vi "NI 9263_task.vi"(8 "error in":errorcluster, 11 "MODULE NAME":string="CDR_AO1") -> (0 "error out":errorcluster, 3 "task out":refnum<k21>)   [LabVIEW 2019]
uses:
  <vilib>/DAQmx/create/channels.llb/DAQmx Create Channel (AO-Voltage-Basic).vi
  <resource>/objmgr/daqmx.rc
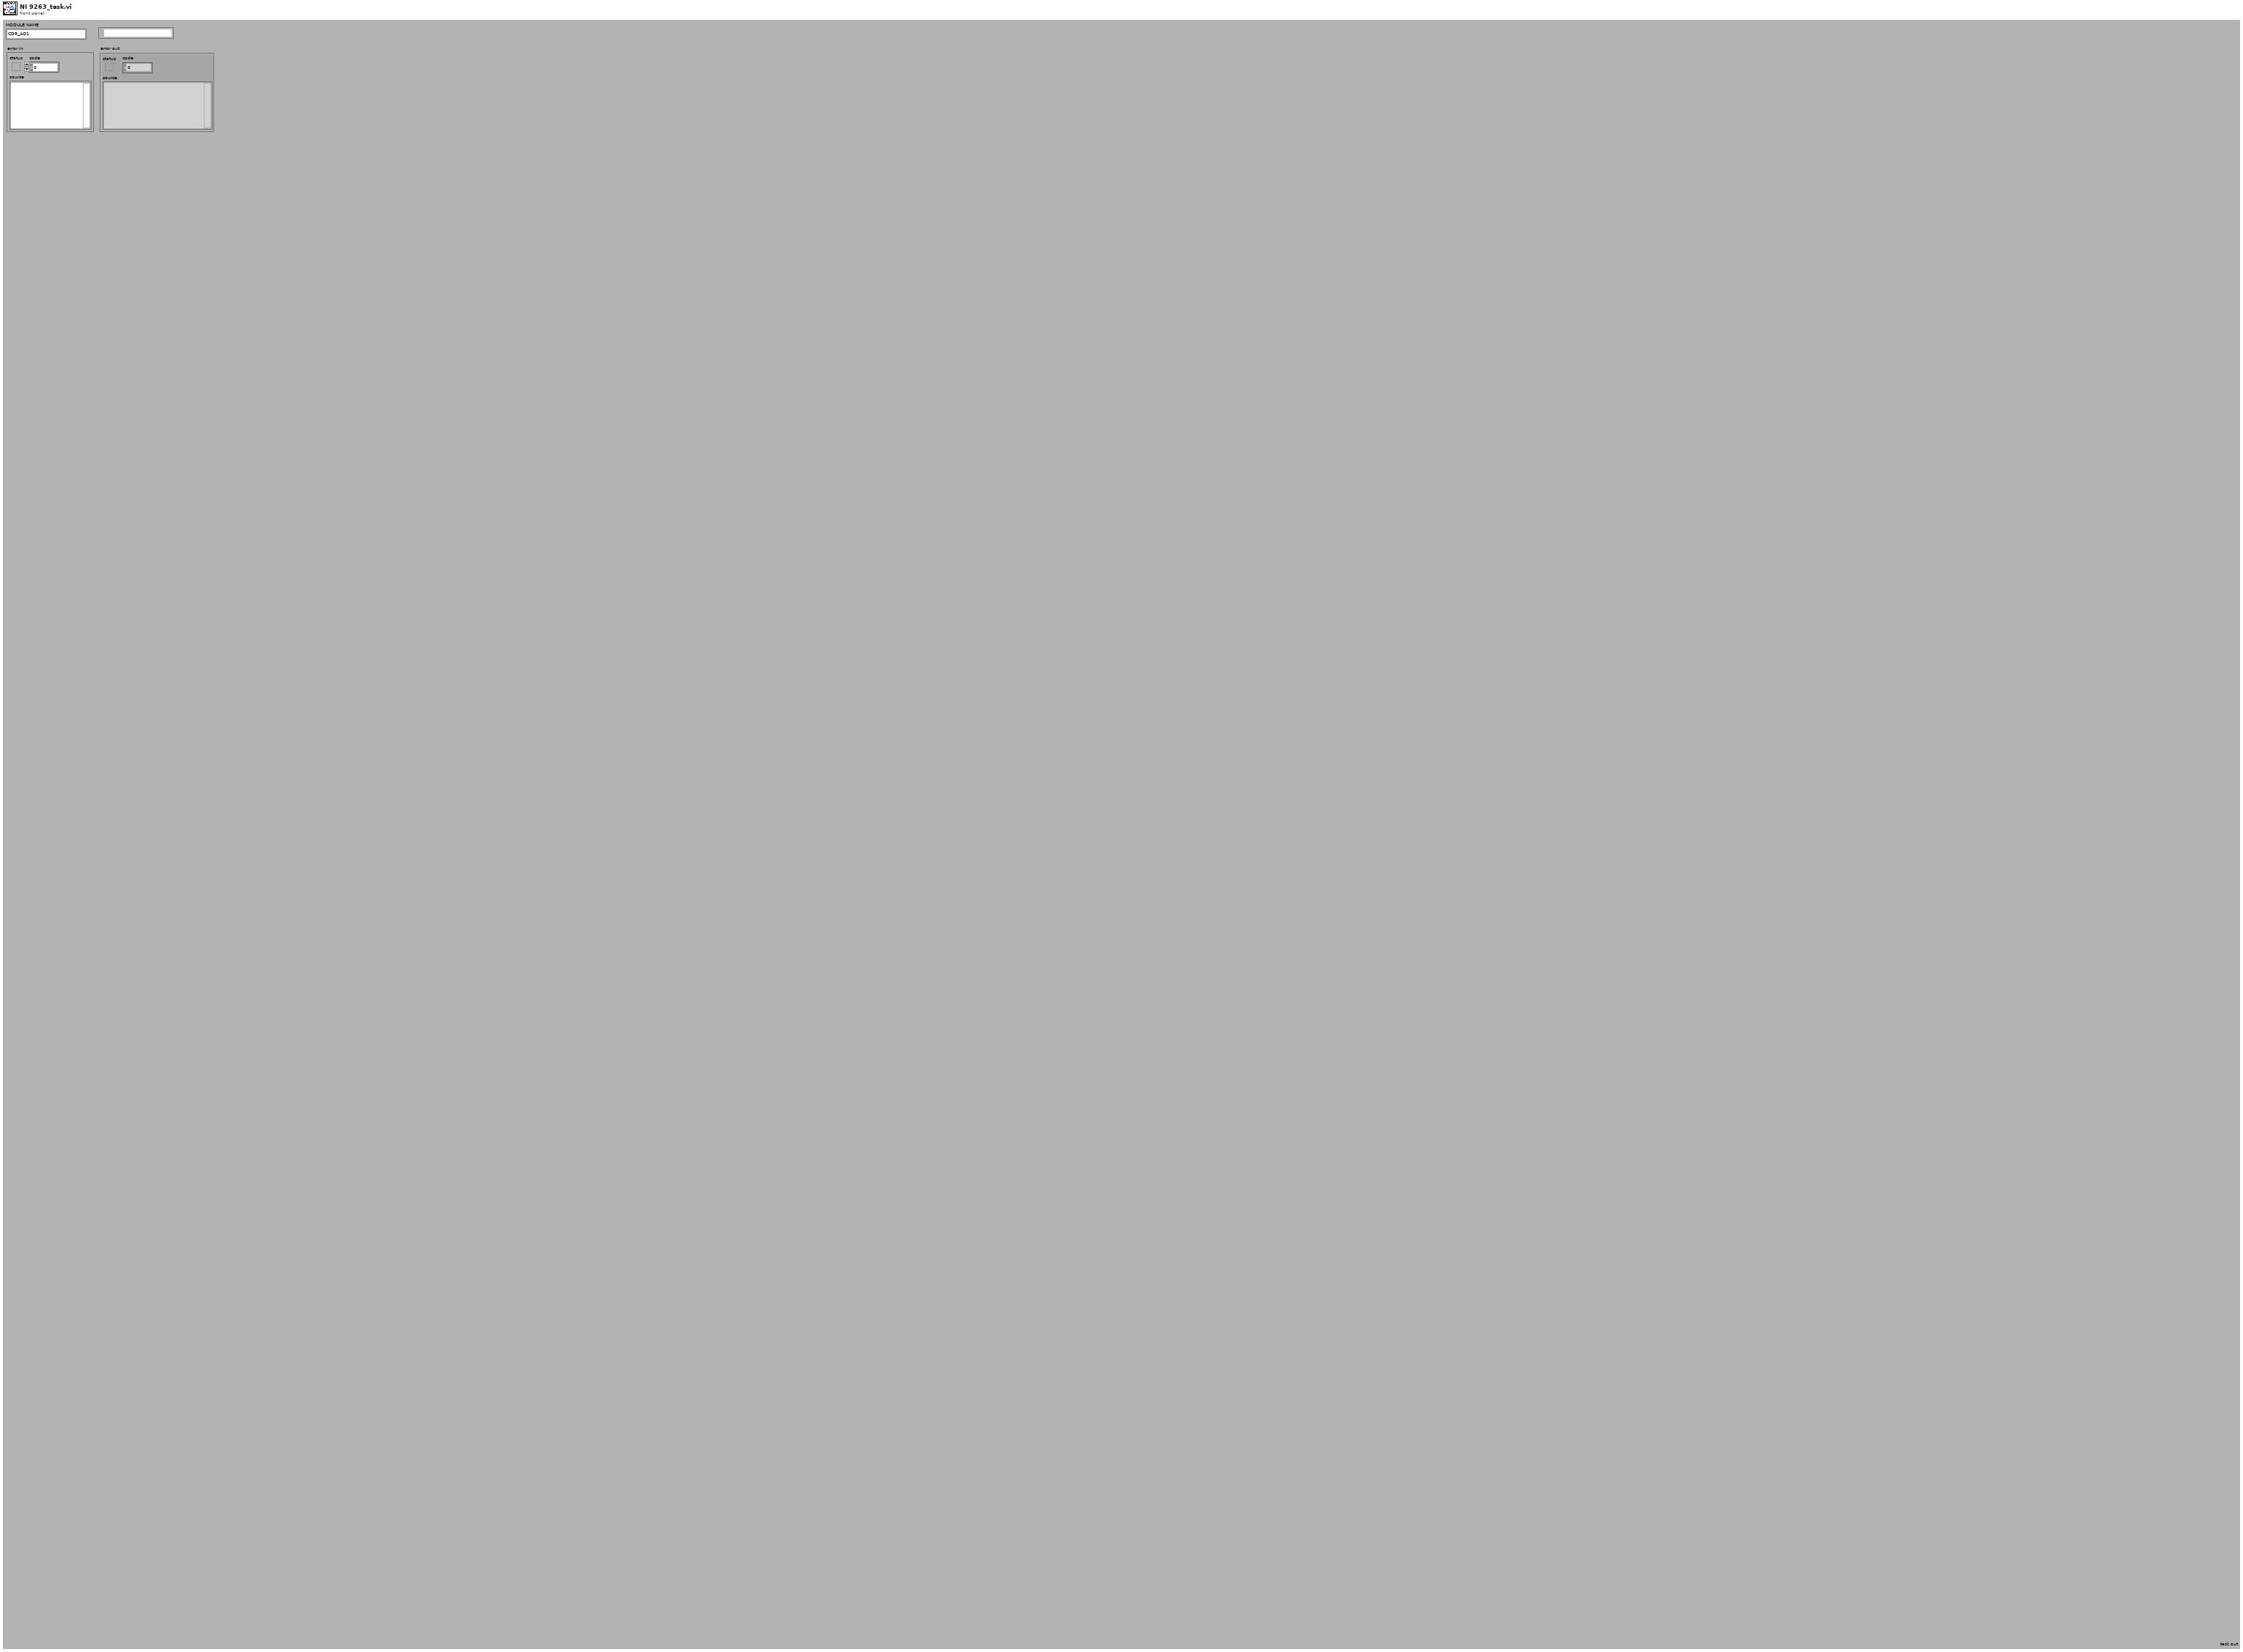
[diagram p1: front panel]
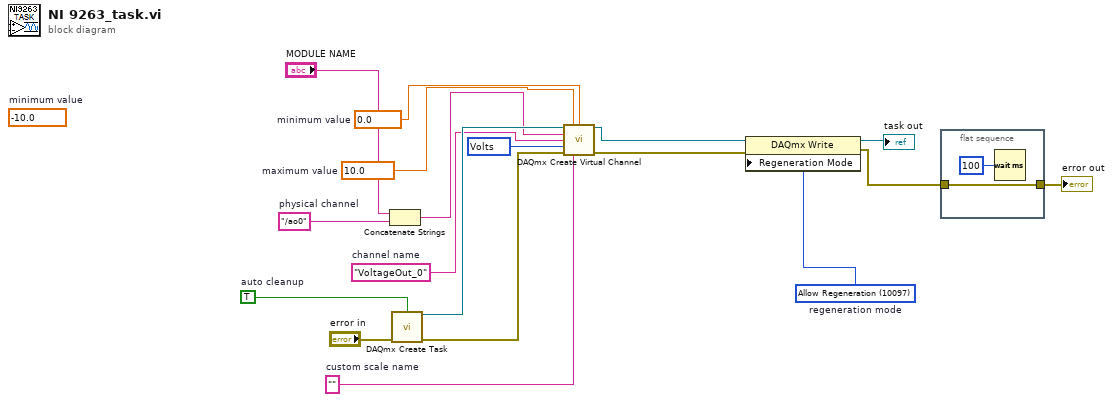
[diagram p0: block diagram]
diagram:
  (unwired) -10.0  # minimum value
  w8 = 10348 items=["Volts"=10348, "From Custom Scale"=10065] ("units")
  w5 = 10097 items=["Allow Regeneration"=10097, "Do Not Allow Regeneration"=10158]  # regeneration mode
  w6 = "VoltageOut_0"  # channel name
  w13 = ""  # custom scale name
  w14 = 0.0  # minimum value
  w15 = 10.0  # maximum value
  w12 = "/ao0"  # physical channel
  w17 = TRUE  # auto cleanup
  n1 = Concatenate Strings("MODULE NAME", w12) -> (w7:string)
  n2 = call <vilib>:"DAQmx Create Task.vi"("auto cleanup"=w17, "error in"="error in") -> ("task out"=w16:refnum<k21>, "error out"=w18:errorcluster)  [unwired: 12 in]
  n3 = call-poly <vilib>:"DAQmx Create Virtual Channel.vi"("task in"=w16, "maximum value"=w15, "minimum value"=w14, "physical channels"=w7, "name to assign"=w6, "units"=w8, "error in"=w18, "custom scale name"=w13) -> ("task out"=w2:refnum<k21>, "error out"=w1:errorcluster)  [unwired: 6 in]
  n4 = property class="DAQmx Write"(reference=w2, error in=w1, "Regeneration Mode"=w5) -> (reference out=→"task out":refnum<k21>, error out=w4:errorcluster)
  n5 = flat-sequence {
    tunnel: [w19] -> w9
    tunnel: w4 -> [w19]
    frame #0 {
      n6 = Wait (ms)(milliseconds to wait=u32 100) -> ()  [unwired: 1 out]
    }
  }
  "error out" <- w9
